vi "dock View in Subpanel.vi"(8 "error in (no error)":errorcluster, 10 "Sub Panel":refnum<vi>, 11 "base view in":refnum<class "base view.lvclass">) -> (0 "error out":errorcluster, 3 "base view out":refnum<class "base view.lvclass">)   [LabVIEW 2022 SP3, in "base view.lvclass"]
uses:
  base view.lvclass
  Accessors/Read View Refnum.vi
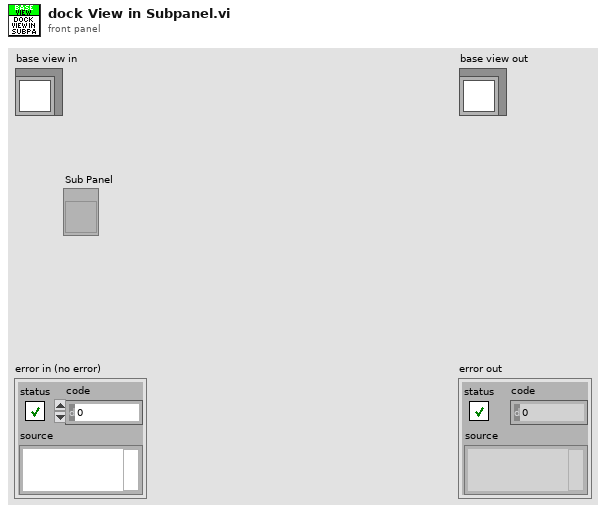
[diagram p1: front panel]
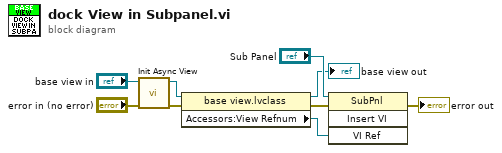
[diagram p0: block diagram]
diagram:
  n1 = call "Init Async View.vi"("error in (no error)"="error in (no error)", "base view in"="base view in") -> ("error out"=w3:errorcluster, "base view out"=w8:refnum<class "base view.lvclass">)  [unwired: 8 in]
  n2 = property class="base view.lvclass"(reference=w8, error in=w3) -> (reference out=→"base view out":refnum<class "base view.lvclass">, error out=w2:errorcluster, "Accessors:View Refnum"=w6:refnum<vi>)
  n3 = invoke class="SubPnl" method="Insert VI"(reference="Sub Panel", error in=w2, "VI Ref"=w6) -> (error out=→"error out":errorcluster)  [unwired: 1 in, 3 out]
